vi "5646R RFSA RFSG Coherency Test.vi"() -> ()   [LabVIEW 2019]
doc: "Use this example to learn the basics of TClk synchronization for RF vector signal analyzers and generators. This example shows how to create NI-RFSA and NI-RFSG sessions and pass them to NI-TClk synchronization functions. It uses NI-TClk to make the NI-RFSA and NI-RFSG start at the same time."
uses:
  <instrlib>/niRFSA/niRFSA.llb/niRFSA Trigger Terminals.ctl
  <instrlib>/niRFSA/niRFSA.llb/niRFSA Acquisition Types.ctl
  <instrlib>/niRFSG/niRFSG.llb/niRFSG Ref Clock Sources.ctl
  <instrlib>/niRFSA/niRFSA.llb/niRFSA Ref Clock Sources.ctl
  <instrlib>/niRFSA/niRFSA.llb/niRFSA Configure Digital Edge Start Trigger.vi
  <instrlib>/niRFSA/niRFSA.llb/niRFSA Fetch IQ (Complex Cluster 1Rec 1Chan).vi
  <instrlib>/niRFSA/niRFSA.llb/niRFSA Get IQ Components (Complex Cluster).vi
panel:
  in  "RX Sample Rate: 100KSps":cluster{"t0":dbl, "dt":dbl, "Y":cdb[]}={"t0"=0.0, "dt"=9.99999999984567e-06, "Y"=array[20000 elements]} {"Y" format="%_2g"; "dt" format="%.6p"; "t0" format="%.6p"}
  in  "RX Sample Rate: 1MSps":cluster{"t0":dbl, "dt":dbl, "Y":cdb[]}={"t0"=0.0, "dt"=9.99999999998778e-07, "Y"=array[20000 elements]} {"Y" format="%_2g"; "dt" format="%.6p"; "t0" format="%.6p"}
  in  "RX Sample Rate: 10MSps":cluster{"t0":dbl, "dt":dbl, "Y":cdb[]}={"t0"=0.0, "dt"=9.999999999998438e-08, "Y"=array[20000 elements]} {"Y" format="%_2g"; "dt" format="%.6p"; "t0" format="%.6p"}
  in  "RX Sample Rate: 100MSps":cluster{"t0":dbl, "dt":dbl, "Y":cdb[]}={"t0"=0.0, "dt"=9.999999999999858e-09, "Y"=array[20000 elements]} {"Y" format="%_2g"; "dt" format="%.6p"; "t0" format="%.6p"}
  in  "data":cluster{"t0":dbl, "dt":dbl, "Y":cdb[]} caption="RX Sample Rate: 100KSps" {"Y" format="%_2g"; "dt" format="%.6p"; "t0" format="%.6p"}
  out "error out":errorcluster {"code" format="%.0x"}
  in  "Remove Frequency Offset":bool
  out "Amplitude Stability":dbl format="%.6p"
  out "Phase Stability":dbl format="%.6p"
  in  "Tab Control":enum32{"     IQ Data", "Magnitude", "Phase"}(tab)
  out "IQ Data":cluster{"t0":dbl, "dt":dbl, "Y":dbl[]}[](graph)
  out "Magnitude":cluster{"t0":dbl, "dt":dbl, "Y":dbl[]}(graph)
  out "Phase":cluster{"t0":dbl, "dt":dbl, "Y":dbl[]}(graph)
  in  "Sync Sample Clock Dist Line":T1="PXI_Trig1"
  in  "RFSA-LO Offset":dbl=10000000.0 caption="LO Offset" format="%.3pHz"
  in  "RFSG-LO Offset":dbl=10000000.0 caption="LO Offset" format="%.3pHz"
  in  "Synchronized Trigger Distribution Line":T1="PXI_Trig0"
  in  "NI-RFSG Device":refnum<k15>="VST-5646R-03"
  in  "RFSG-Power Level (dBm)":dbl=-20.0 caption="Power Level (dBm)" format="%.2f"
  in  "RFSG-Frequency (Hz)":dbl=1000000000.0 caption="Frequency (Hz)" format="%.6p"
  in  "NI-RFSA Device":refnum<k15>="VST-5646R-03"
  in  "RFSA-Number of Samples":i64=100 caption="Number of Samples"
  in  "RFSA-IQ rate (S/s)":dbl=1000000.0 caption="IQ rate (S/s)" format="%#_6p"
  in  "RFSA-Carrier Frequency (Hz)":dbl=1000000000.0 caption="IQ Carrier Frequency (Hz)" format="%_6p"
  in  "RFSA-Reference Level (dBm)":dbl=-20.0 caption="Reference Level (dBm)" format="%.2f"
  # "NI-RFSG Settings"
  # "NI-RFSA Settings"
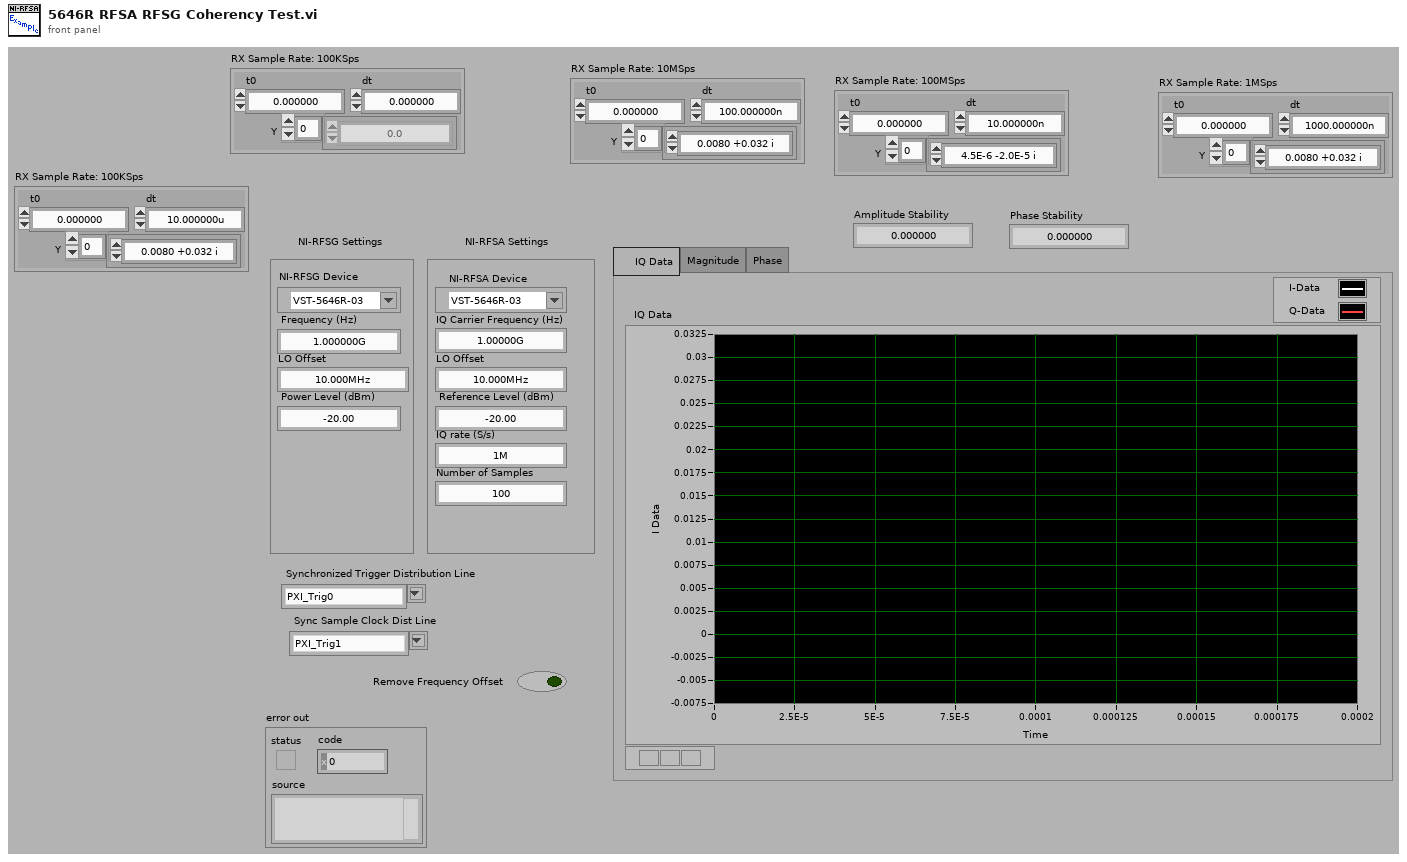
[diagram p1: front panel]
types:
  T1 = typedef "niRFSA Trigger Terminals.ctl" = string
  T2 = typedef "niRFSA Ref Clock Sources.ctl" = string
  T3 = typedef "niRFSG Ref Clock Sources.ctl" = string
  T4 = typedef "niRFSA Acquisition Types.ctl" = i32
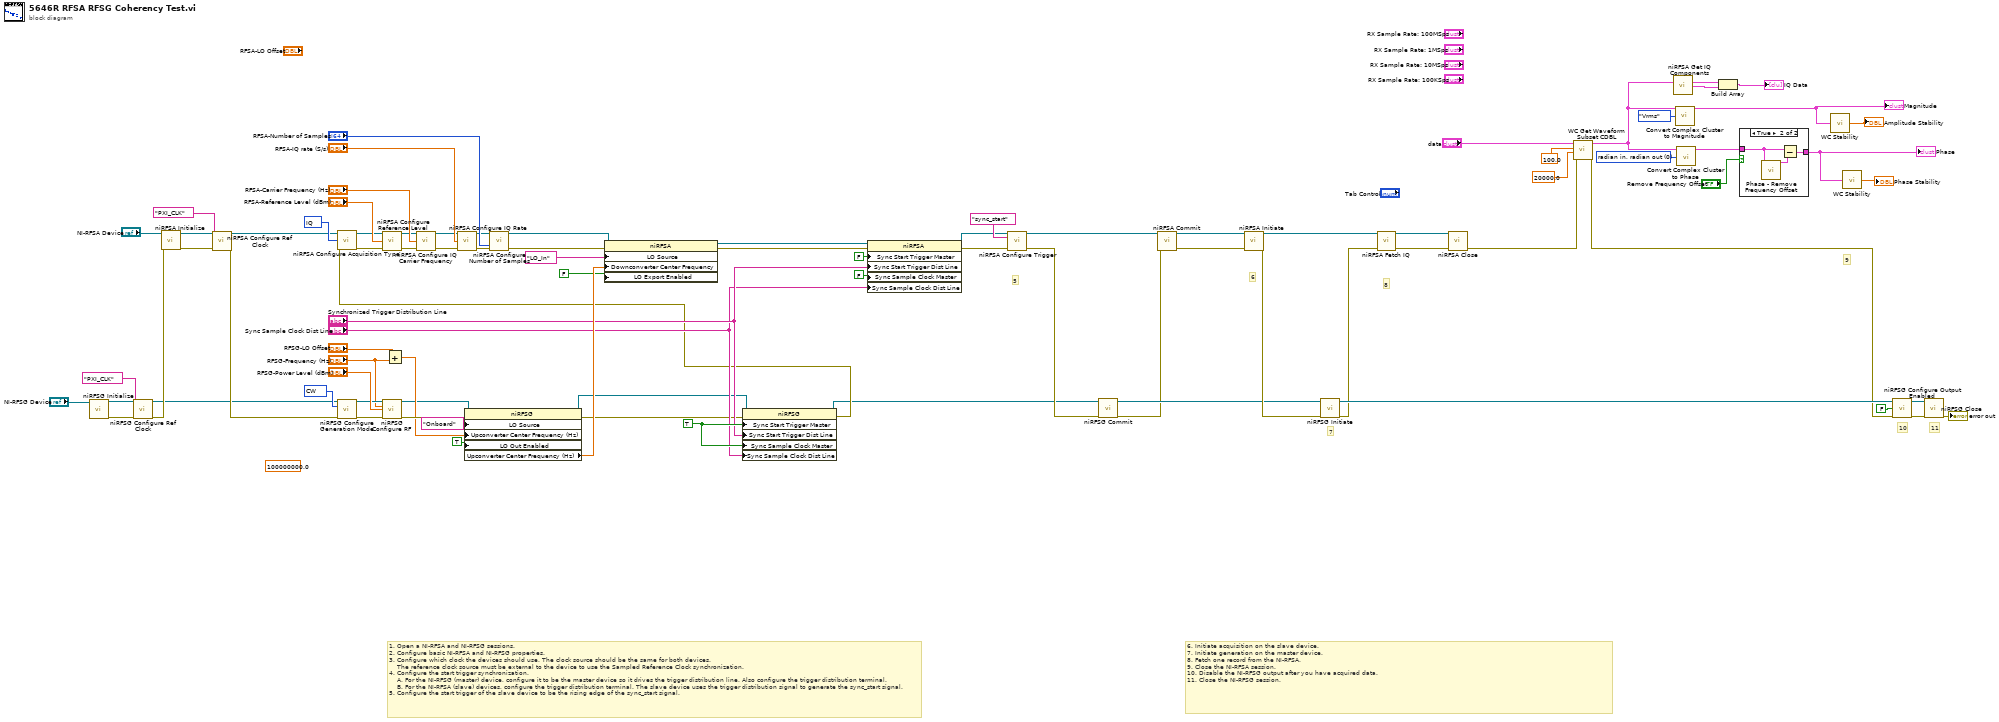
[diagram p0: block diagram]
diagram:
  (unwired) 100000000.0 ("Arb:IQ Rate (S/s)")
  w42 = 0 items=["radian in, radian out", "radian in, degree out", "degree in, degree out", "degree in, radian out"] ("phase unit")
  w56 = TRUE ("Device Specific:5644R and 5645R:Triggers:Sync Script Trigger Master")
  w70 = T4 100 items=["IQ"=100, "Spectrum"=101] ("acquisition type")
  w87 = 1000 items=["CW"=1000, "Arb Waveform"=1001, "Script"=1002] ("generation mode")
  # "7"
  # "9"
  # "6. Initiate acquisition on the slave device.\n7. Initiate generation on the master device.\n8. Fetch one record from the NI-RFSA.\n9. Close the NI-RFSA session.\n10. Disable the NI-RFSG output after you have acquired data.\n11. Close the NI-RFSG session."
  # "6"
  # "5"
  # "8"
  # "11"
  # "10"
  # "1. Open a NI-RFSA and NI-RFSG sessions.\n2. Configure basic NI-RFSA and NI-RFSG properties.\n3. Configure which clock the devices should use. The clock source should be the same for both devices.\n    The reference clock source must be external to the device to use the Sampled Reference Clock synchronization.\n4. Configure the start trigger synchronization.\n    A. For the NI-RFSG (master) device, configure it to be the master device so it drives the trigger distribution line. Also configure the trigger distribution terminal.\n    B. For the NI-RFSA (slave) devices, configure the trigger distribution terminal. The slave device uses the trigger distribution signal to generate the sync_start signal.\n5. Configure the start trigger of the slave device to be the rising edge of the sync_start signal."
  n1 = call <instrlib>:"niRFSG Initialize.vi"("resource name"="NI-RFSG Device") -> ("instrument handle"=w13:refnum<k15>, "error out"=w25:errorcluster)  [unwired: 3 in, 10 out]
  n2 = call <instrlib>:"niRFSG Configure Ref Clock.vi"("instrument handle"=w13, "ref clock source"=T3 "PXI_CLK", "error in"=w25) -> ("instrument handle out"=w12:refnum<k15>, "error out"=w24:errorcluster)  [unwired: 1 in, 10 out]
  n3 = call <instrlib>:"niRFSA Initialize.vi"("resource name"="NI-RFSA Device", "error in"=w24) -> ("instrument handle out"=w14:refnum<k15>, "error out"=w23:errorcluster)  [unwired: 2 in, 10 out]
  n4 = call <instrlib>:"niRFSA Configure Ref Clock.vi"("instrument handle"=w14, "clock source"=T2 "PXI_CLK", "error in"=w23) -> ("instrument handle out"=w15:refnum<k15>, "error out"=w22:errorcluster)  [unwired: 1 in, 10 out]
  n5 = call <instrlib>:"niRFSG Configure Generation Mode.vi"("instrument handle"=w12, "generation mode"=w87, "error in"=w22) -> ("instrument handle out"=w63:refnum<k15>, "error out"=w64:errorcluster)  [unwired: 11 out]
  n6 = call <instrlib>:"niRFSG Configure RF.vi"("instrument handle"=w63, "frequency (Hz)"="RFSG-Frequency (Hz)", "power level (dBm)"="RFSG-Power Level (dBm)", "error in"=w64) -> ("instrument handle out"=w55:refnum<k15>, "error out"=w59:errorcluster)  [unwired: 10 out]
  n7 = Add(x="RFSG-LO Offset", y="RFSG-Frequency (Hz)") -> (x+y=w58:dbl)
  n8 = property class="niRFSG"(reference=w55, error in=w59, "LO Source"="Onboard" ("Device Specific:Vector Signal Transceiver:Signal Path:LO Source"), "Upconverter Center Frequency (Hz)"=w58, "LO Out Enabled"=TRUE ("RF:LO Out Enabled")) -> (reference out=w20:refnum<k15>, error out=w21:errorcluster, "Upconverter Center Frequency (Hz)"=w52:dbl)
  n9 = property class="niRFSG"(reference=w20, error in=w21, "Sync Start Trigger Master"=w56, "Sync Start Trigger Dist Line"="Synchronized Trigger Distribution Line", "Sync Sample Clock Master"=w56, "Sync Sample Clock Dist Line"="Sync Sample Clock Dist Line") -> (reference out=w8:refnum<k15>, error out=w19:errorcluster)
  n10 = call <instrlib>:"niRFSA Configure Acquisition Type.vi"("instrument handle"=w15, "acquisition type"=w70, "error in"=w19) -> ("instrument handle out"=w78:refnum<k15>, "error out"=w77:errorcluster)  [unwired: 11 out]
  n11 = call <instrlib>:"niRFSA Configure Reference Level.vi"("instrument handle"=w78, "reference level (dBm)"="RFSA-Reference Level (dBm)", "error in"=w77) -> ("instrument handle out"=w76:refnum<k15>, "error out"=w75:errorcluster)  [unwired: 11 out]
  n12 = call <instrlib>:"niRFSA Configure IQ Carrier Frequency.vi"("instrument handle"=w76, "carrier frequency"="RFSA-Carrier Frequency (Hz)", "error in"=w75) -> ("instrument handle out"=w74:refnum<k15>, "error out"=w73:errorcluster)  [unwired: 11 out]
  n13 = call <instrlib>:"niRFSA Configure IQ Rate.vi"("instrument handle"=w74, "IQ rate (S/s)"="RFSA-IQ rate (S/s)", "error in"=w73) -> ("instrument handle out"=w72:refnum<k15>, "error out"=w71:errorcluster)  [unwired: 11 out]
  n14 = call <instrlib>:"niRFSA Configure Number of Samples.vi"("instrument handle"=w72, "samples per record"="RFSA-Number of Samples", "error in"=w71) -> ("instrument handle out"=w44:refnum<k15>, "error out"=w53:errorcluster)  [unwired: 1 in, 10 out]
  n15 = property class="niRFSA"(reference=w44, error in=w53, "LO Source"="LO_In" ("Signal Path:LO Source"), "Downconverter Center Frequency"=w52, "LO Export Enabled"=FALSE ("Signal Path:LO Export Enabled")) -> (reference out=w17:refnum<k15>, error out=w18:errorcluster)
  n16 = property class="niRFSA"(reference=w17, error in=w18, "Sync Start Trigger Master"=FALSE ("Device Specific:5644R and 5645R:Triggers:Synchronization:Sync Start Trigger Master"), "Sync Start Trigger Dist Line"="Synchronized Trigger Distribution Line", "Sync Sample Clock Master"=FALSE ("Device Specific:5644R and 5645R:Triggers:Synchronization:Sync Start Trigger Master"), "Sync Sample Clock Dist Line"="Sync Sample Clock Dist Line") -> (reference out=w47:refnum<k15>, error out=w48:errorcluster)
  n17 = call-poly <instrlib>:"niRFSA Configure Trigger.vi"("instrument handle"=w47, "source"=T1 "sync_start", "error in"=w48) -> ("instrument handle out"=w5:refnum<k15>, "error out"=w9:errorcluster)  [unwired: 11 in]
  n18 = call <instrlib>:"niRFSG Commit.vi"("instrument handle"=w8, "error in"=w9) -> ("instrument handle out"=w7:refnum<k15>, "error out"=w6:errorcluster)  [unwired: 12 in]
  n19 = call <instrlib>:"niRFSA Commit.vi"("instrument handle"=w5, "error in"=w6) -> ("instrument handle out"=w4:refnum<k15>, "error out"=w3:errorcluster)  [unwired: 12 in]
  n20 = call <instrlib>:"niRFSA Initiate.vi"("instrument handle"=w4, "error in"=w3) -> ("instrument handle out"=w67:refnum<k15>, "error out"=w16:errorcluster)  [unwired: 12 in]
  n21 = call <instrlib>:"niRFSG Initiate.vi"("instrument handle"=w7, "error in"=w16) -> ("instrument handle out"=w68:refnum<k15>, "error out"=w65:errorcluster)  [unwired: 12 in]
  n22 = call-poly <instrlib>:"niRFSA Fetch IQ.vi"("instrument handle"=w67, "error in"=w65) -> ("instrument handle out"=w29:refnum<k15>, "error out"=w28:errorcluster)  [unwired: 3 in, 9 out]
  n23 = call <instrlib>:"niRFSA Close.vi"("instrument handle"=w29, "error in"=w28) -> ("error out"=w27:errorcluster)  [unwired: 13 out]
  n24 = call "WC Get Waveform Subset CDBL.vi"("error in (no error)"=w27, "duration"=20000.0, "start samples/time"=100.0, "Waveform In"="data") -> ("error out"=w26:errorcluster, "Waveform Out"=w39:cluster{"t0":dbl, "dt":dbl, "Y":cdb[]})  [unwired: 2 in, 2 out]
  n25 = call-poly <instrlib>:"niRFSA Get IQ Components.vi"("data"=w39) -> ("I"=w41:cluster{"t0":dbl, "dt":dbl, "Y":dbl[]}, "Q"=w40:cluster{"t0":dbl, "dt":dbl, "Y":dbl[]})  [unwired: 1 in, 12 out]
  n26 = call "Convert Complex Cluster to Magnitude.vi"("IQ data (complex) In"=w39, "Public.Units"=enum8{"Vrms", "dBm"}."Vrms") -> ("Magnitude Out"=w31:cluster{"t0":dbl, "dt":dbl, "Y":dbl[]})  [unwired: 12 in, 1 out]
  "Magnitude" <- w31
  n27 = call "Convert Complex Cluster to Phase.vi"("IQ data (complex) In"=w39, "phase unit"=w42) -> ("Phase Out"=w38:cluster{"t0":dbl, "dt":dbl, "Y":dbl[]})  [unwired: 12 in, 1 out]
  n28 = Build Array(w41, w40) -> (→"IQ Data":cluster{"t0":dbl, "dt":dbl, "Y":dbl[]}[])
  n29 = case shown="True" "Remove Frequency Offset" {
    tunnel: w38 -> [w89 w91]
    tunnel: [w89 w90] -> w30
    frame False {
    }
    frame True {
      n30 = call "Phase - Remove Frequency Offset.vi"("Phase In"=w91) -> ("Phase Out"=w92:cluster{"t0":dbl, "dt":dbl, "Y":dbl[]})  [unwired: 13 in, 1 out]
      n31 = Subtract(x=w91, y=w92) -> (x-y=w90:cluster{"t0":dbl, "dt":dbl, "Y":dbl[]})
    }
  }
  "Phase" <- w30
  n32 = call "WC Stability.vi"("Data In"=w31) -> ("Stability"=→"Amplitude Stability":dbl)  [unwired: 4 in]
  n33 = call "WC Stability.vi"("Data In"=w30) -> ("Stability"=→"Phase Stability":dbl)  [unwired: 4 in]
  n34 = call <instrlib>:"niRFSG Configure Output Enabled.vi"("instrument handle"=w68, "output enabled"=FALSE, "error in"=w26) -> ("instrument handle out"=w86:refnum<k15>, "error out"=w85:errorcluster)  [unwired: 11 out]
  n35 = call <instrlib>:"niRFSG Close.vi"("instrument handle"=w86, "error in"=w85) -> ("error out"=→"error out":errorcluster)  [unwired: 13 out]
